vi "Generate Rectangle Seq Img Core.vi"(6 "TDMS file path & name":path=path "C:/Users/Theo/Desktop/Datasets/140401_17_44_08-rig 3 debugging/Functional imaging TDMS data files/001.tdms", 7 "Channel to process":enum16{"Red", "Green"}(ring), 8 "error in (no error)":errorcluster, 9 "<Vol images/video folder>":path, 10 "All header parameters":T1={"LOGIN"={"User"="Olympus  20X", "Profile"="", "Software Version"="", "Experiment Date Time"=timestamp(0 s since 1904-01-01)}, "GLOBAL PARAMETERS"={"MicroscopeID"="", "Microscope Type"="", "Objective"="", "Field of View (um)"=0.0, "Fill time (us)"=0.0, "Experiment Type"=enum."In vivo", "Stimuli Trigger"=FALSE, "Speed Logging"=FALSE}, "IMAGING MODES"={"Time Series"=FALSE, "Motor Zstack"=FALSE, "AOL Zstack"=FALSE, "Functional Imaging"=FALSE, "Volume Imaging"=FALSE}, "TIME SERIES"={"Basic Image meta data"={"Wavelength (nm)"=0.0, "# averaged frames"=0.0, "laser power (%)"=0.0, "Pockels"=0.0, "pixel dwell time (us)"=0.0, "pmt 1"=0.0, "pmt 2"=0.0, "back apperture"=0.0, "zoom"=0.0, "field of view"=0.0, "Frame Size"=0, "AOL x centre"=200.0, "AOL y centre"=0.0, "Stage x position"=0.0, "Stage y position"=0.0, "Stage z position"=0.0}, "AOL z"=0.0}, "MOTOR Z-STACK "={"Hdr Basic Image meta data"={"Wavelength (nm)"=0.0, "# averaged frames"=0.0, "laser power (%)"=0.0, "Pockels"=0.0, "pixel dwell time (us)"=0.0, "pmt 1"=0.0, "pmt 2"=0.0, "back apperture"=0.0, "zoom"=0.0, "field of view"=0.0, "Frame Size"=0, "AOL x centre"=0.0, "AOL y centre"=0.0, "Stage x position"=0.0, "Stage y position"=0.0, "Stage z position"=0.0}, "Z Start"=0.0, "Z Stop"=0.0, "No of Planes"=0}, "AOL Z-STACK"={"Hdr Basic Image meta data"={"Wavelength (nm)"=0.0, "# averaged frames"=0.0, "laser power (%)"=0.0, "Pockels"=0.0, "pixel dwell time (us)"=0.0, "pmt 1"=0.0, "pmt 2"=0.0, "back apperture"=0.0, "zoom"=0.0, "field of view"=0.0, "Frame Size"=0, "AOL x centre"=0.0, "AOL y centre"=0.0, "Stage x position"=0.0, "Stage y position"=0.0, "Stage z position"=0.0}, "Z Start"=0.0, "Z Stop"=0.0, "No of Planes"=0}, "FUNCTIONAL IMAGING"={"Functional Mode"=enum."Point", "Pockels Modulation"=FALSE, "Number of pois"=0.0, "Number of miniscans"=0.0, "Number of cycles"=0.0, "Number of trials"=0.0, "Miniscan dwell time per pixel (us)"=0.0, "Number of pixels in miniscan"=0.0, "poi dwell time"=0.0, "Rectangle ROI length"=0.0, "Rectangle ROI height"=0.0, "AOL Mode"=enum."Raster", "Plane Mode"=0, "video length (sec)"=0.0, "Frame rate (fps)"=0.0, "Stimuli Timing (usec)"=0.0, "Acquisition Length"=0.0, "Basic Image meta data"={"Wavelength (nm)"=0.0, "# averaged frames"=0.0, "laser power (%)"=0.0, "Pockels"=0.0, "pixel dwell time (us)"=0.0, "pmt 1"=0.0, "pmt 2"=0.0, "back apperture"=0.0, "zoom"=0.0, "field of view"=0.0, "Frame Size"=0, "AOL x centre"=0.0, "AOL y centre"=0.0, "Stage x position"=0.0, "Stage y position"=0.0, "Stage z position"=0.0}, "Z Start (um)"=0.0, "Z Stop (um)"=0.0}, "VOLUME IMAGING"={"Functional Mode"=enum."Point", "Pockels Modulation"=FALSE, "Number of pois"=0.0, "Number of miniscans"=0.0, "Number of cycles"=0.0, "Number of trials"=0.0, "Miniscan dwell time per pixel (us)"=0.0, "Number of pixels in miniscan"=0.0, "poi dwell time"=0.0, "Rectangle ROI length"=0.0, "Rectangle ROI height"=0.0, "AOL Mode"=enum."Raster", "Plane Mode"=0, "video length (sec)"=0.0, "Frame rate (fps)"=0.0, "Stimuli Timing (usec)"=0.0, "Acquisition Length"=0.0, "Basic Image meta data"={"Wavelength (nm)"=0.0, "# averaged frames"=0.0, "laser power (%)"=0.0, "Pockels"=0.0, "pixel dwell time (us)"=0.0, "pmt 1"=0.0, "pmt 2"=0.0, "back apperture"=0.0, "zoom"=0.0, "field of view"=0.0, "Frame Size"=0, "AOL x centre"=0.0, "AOL y centre"=0.0, "Stage x position"=0.0, "Stage y position"=0.0, "Stage z position"=0.0}, "Z Start (um)"=0.0, "Z Stop (um)"=0.0}, "CALIBRATION"={"Pockels Calibration File"=path "", "Calibration_ini file"=path "", "Setup_ini file"=path ""}, "STATISTICS"={"Z-stack duration (sec)"=0.0, "Number of acquired data-points"=0.0, "Acquisition time (ms)"=0.0, "Number of acquired frames"=0.0, "Intertrial times"=[]}, "BIOLOGY INFORMATION"={"Animal Code or Name"="", "Animal DoB"="", "Animal Age"="", "Animal Sex"="", "Animal Weight"="", "Date of Injection"="", "Date of Implant"="", "Site of Injection"="", "Animal Ear Notch"="", "AAV constructs"="", "Genetic background"="", "Optical reporter"="", "Region of brain imaged"="", "Other \ncomments"=""}} {"VOLUME IMAGING"."Plane Mode" items=["XY Plane", "XZ Plane", "YZ Plane", "arbitraryplane"]; "VOLUME IMAGING"."Basic Image meta data"."Frame Size" items=["100X100"=100, "128X128"=128, "200X200"=200, "256X256"=256, "512X512"=512, "1024x1024"=1024, "2048x2048"=2048]; "AOL Z-STACK"."Hdr Basic Image meta data"."Frame Size" items=["100X100"=100, "128X128"=128, "200X200"=200, "256X256"=256, "512X512"=512, "1024x1024"=1024, "2048x2048"=2048]; "MOTOR Z-STACK"."Hdr Basic Image meta data"."Frame Size" items=["100X100"=100, "128X128"=128, "200X200"=200, "256X256"=256, "512X512"=512, "1024x1024"=1024, "2048x2048"=2048]; "FUNCTIONAL IMAGING"."Plane Mode" items=["XY Plane", "XZ Plane", "YZ Plane", "arbitraryplane"]; "FUNCTIONAL IMAGING"."Basic Image meta data"."Frame Size" items=["100X100"=100, "128X128"=128, "200X200"=200, "256X256"=256, "512X512"=512, "1024x1024"=1024, "2048x2048"=2048]; "TIME SERIES"."Basic Image meta data"."Frame Size" items=["100X100"=100, "128X128"=128, "200X200"=200, "256X256"=256, "512X512"=512, "1024x1024"=1024, "2048x2048"=2048]}, 11 "tdms file ref":refnum<k34>) -> (0 "error out":errorcluster, 3 "tdms file out":refnum<k34>)   [LabVIEW 2017]
uses:
  User Interface/Visualisation/Functional Imaging Viewer/SubVIs/Experiment header interface/Typedefs/Header parameters cluster-ALL.ctl
  User Interface/Visualisation/Functional Imaging Viewer/SubVIs/Experiment header interface/Typedefs/Header subclusters/Header params -Login.ctl
  User Interface/Visualisation/Functional Imaging Viewer/SubVIs/Experiment header interface/Typedefs/Header subclusters/Header params-Global Parameters.ctl
  User Interface/Misc/Experiment Type.ctl
  User Interface/Visualisation/Functional Imaging Viewer/SubVIs/Experiment header interface/Typedefs/Header subclusters/Header params-Imaging Modes.ctl
  User Interface/Visualisation/Functional Imaging Viewer/SubVIs/Experiment header interface/Typedefs/Header subclusters/Header params-Time Series.ctl
  User Interface/Visualisation/Functional Imaging Viewer/SubVIs/Experiment header interface/Typedefs/Header subclusters/Header params-Basic image meta data.ctl
  Typedefs/Frame Size.ctl
  User Interface/Visualisation/Functional Imaging Viewer/SubVIs/Experiment header interface/Typedefs/Header subclusters/Header params-Motor Z-stack.ctl
  User Interface/Visualisation/Functional Imaging Viewer/SubVIs/Experiment header interface/Typedefs/Header subclusters/Header params-AOL Z-stack.ctl
  User Interface/Visualisation/Functional Imaging Viewer/SubVIs/Experiment header interface/Typedefs/Header subclusters/Header params-Functional Imaging.ctl
  Typedefs/Functional Mode.ctl
  Typedefs/AOL modes.ctl
  Typedefs/Plane Mode.ctl
  User Interface/Visualisation/Functional Imaging Viewer/SubVIs/Experiment header interface/Typedefs/Header subclusters/Header params-Calibration Setup.ctl
  User Interface/Visualisation/Functional Imaging Viewer/SubVIs/Experiment header interface/Typedefs/Header subclusters/Header params-statistics.ctl
  User Interface/Misc/Biology Information.ctl
  Typedefs/Channel Selector.ctl
  <vilib>/vision/NI_Vision_Development_Module.lvlib
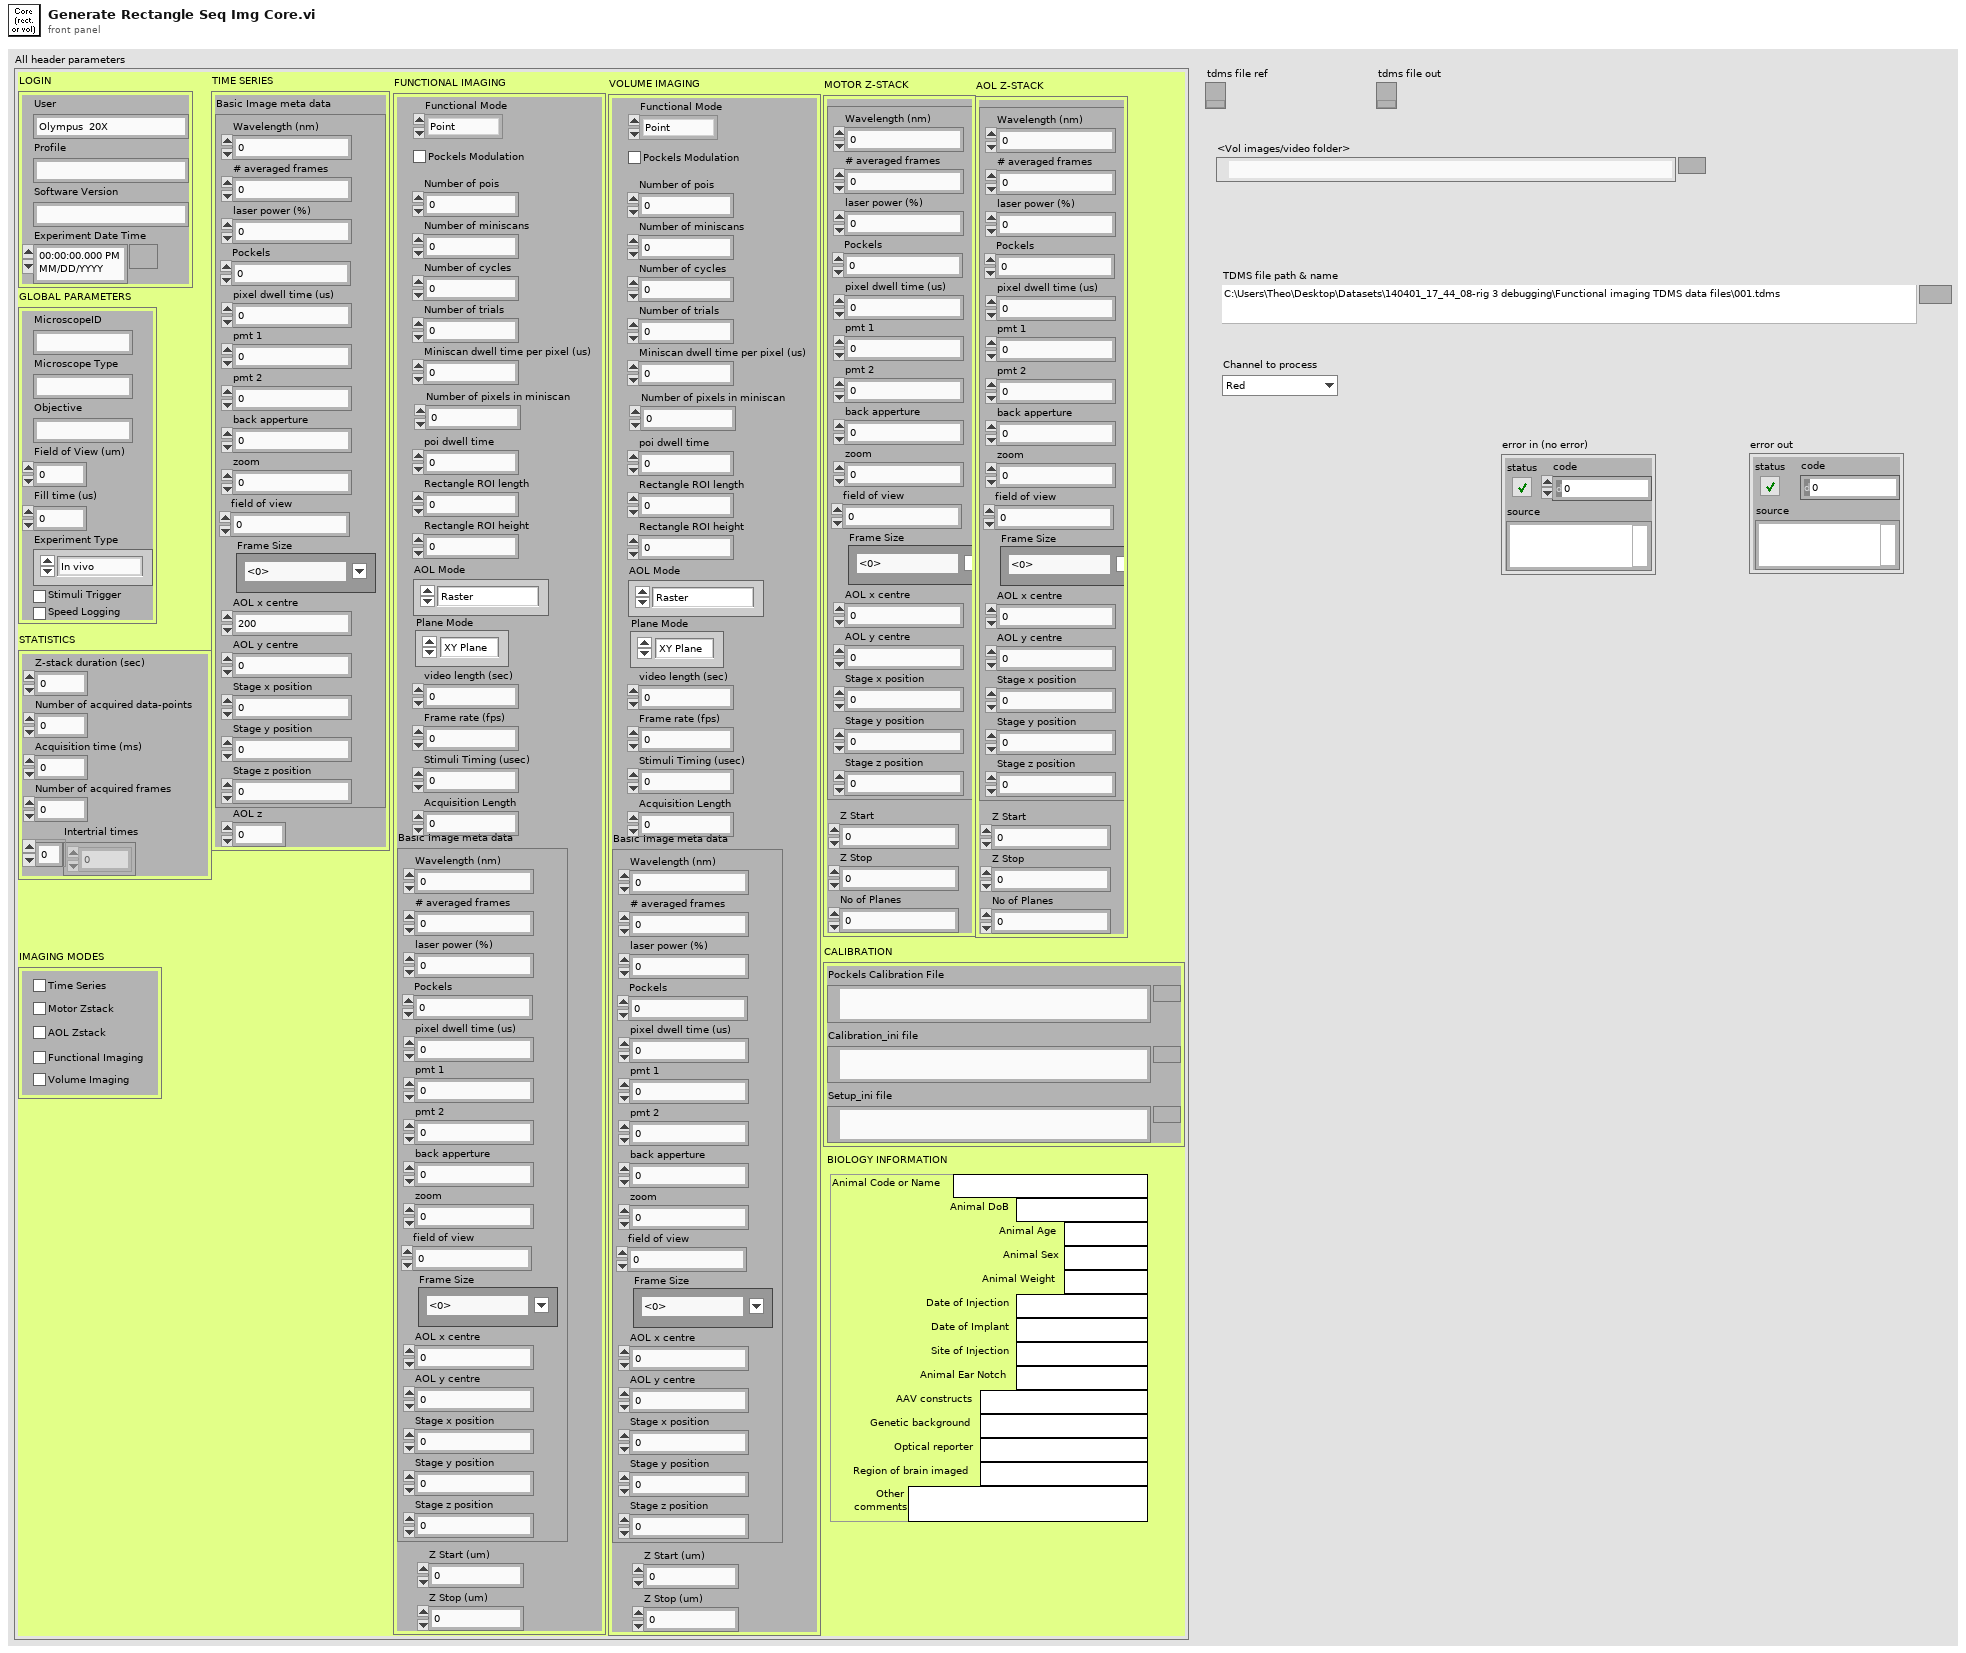
[diagram p1: front panel]
types:
  T1 = typedef "Header parameters cluster-ALL.ctl" = cluster{"LOGIN":T2, "GLOBAL PARAMETERS":T3, "IMAGING MODES":T5, "TIME SERIES":T6, "MOTOR Z-STACK ":T9, "AOL Z-STACK":T10, "FUNCTIONAL IMAGING":T11, "VOLUME IMAGING":T11, "CALIBRATION":T15, "STATISTICS":T16, "BIOLOGY INFORMATION":T17}
  T2 = typedef "Header params -Login.ctl" = cluster{"User":string, "Profile":string, "Software Version":string, "Experiment Date Time":timestamp}
  T3 = typedef "Header params-Global Parameters.ctl" = cluster{"MicroscopeID":string, "Microscope Type":string, "Objective":string, "Field of View (um)":dbl, "Fill time (us)":dbl, "Experiment Type":T4, "Stimuli Trigger":bool, "Speed Logging":bool}
  T4 = typedef "Experiment Type.ctl" = enum16{"In vivo", "In vitro", "Testing", "Calibration", "Other"}
  T5 = typedef "Header params-Imaging Modes.ctl" = cluster{"Time Series":bool, "Motor Zstack":bool, "AOL Zstack":bool, "Functional Imaging":bool, "Volume Imaging":bool}
  T6 = typedef "Header params-Time Series.ctl" = cluster{"Basic Image meta data":T7, "AOL z":dbl}
  T7 = typedef "Header params-Basic image meta data.ctl" = cluster{"Wavelength (nm)":dbl, "# averaged frames":dbl, "laser power (%)":dbl, "Pockels":dbl, "pixel dwell time (us)":dbl, "pmt 1":dbl, "pmt 2":dbl, "back apperture":dbl, "zoom":dbl, "field of view":dbl, "Frame Size":T8, "AOL x centre":dbl, "AOL y centre":dbl, "Stage x position":dbl, "Stage y position":dbl, "Stage z position":dbl}
  T8 = typedef "Frame Size.ctl" = u16
  T9 = typedef "Header params-Motor Z-stack.ctl" = cluster{"Hdr Basic Image meta data":T7, "Z Start":dbl, "Z Stop":dbl, "No of Planes":i32}
  T10 = typedef "Header params-AOL Z-stack.ctl" = cluster{"Hdr Basic Image meta data":T7, "Z Start":dbl, "Z Stop":dbl, "No of Planes":i32}
  T11 = typedef "Header params-Functional Imaging.ctl" = cluster{"Functional Mode":T12, "Pockels Modulation":bool, "Number of pois":dbl, "Number of miniscans":dbl, "Number of cycles":dbl, "Number of trials":dbl, "Miniscan dwell time per pixel (us)":dbl, "Number of pixels in miniscan":dbl, "poi dwell time":dbl, "Rectangle ROI length":dbl, "Rectangle ROI height":dbl, "AOL Mode":T13, "Plane Mode":T14, "video length (sec)":dbl, "Frame rate (fps)":dbl, "Stimuli Timing (usec)":dbl, "Acquisition Length":dbl, "Basic Image meta data":T7, "Z Start (um)":dbl, "Z Stop (um)":dbl}
  T12 = typedef "Functional Mode.ctl" = enum16{"Point", "Line", "Patch", "Plane", "Volume"}
  T13 = typedef "AOL modes.ctl" = enum16{"Raster", "Structural", "Pointing", "Mini Scan", "Alignment"}
  T14 = typedef "Plane Mode.ctl" = u16
  T15 = typedef "Header params-Calibration Setup.ctl" = cluster{"Pockels Calibration File":path, "Calibration_ini file":path, "Setup_ini file":path}
  T16 = typedef "Header params-statistics.ctl" = cluster{"Z-stack duration (sec)":dbl, "Number of acquired data-points":dbl, "Acquisition time (ms)":dbl, "Number of acquired frames":dbl, "Intertrial times":dbl[]}
  T17 = typedef "Biology Information.ctl" = cluster{"Animal Code or Name":string, "Animal DoB":string, "Animal Age":string, "Animal Sex":string, "Animal Weight":string, "Date of Injection":string, "Date of Implant":string, "Site of Injection":string, "Animal Ear Notch":string, "AAV constructs":string, "Genetic background":string, "Optical reporter":string, "Region of brain imaged":string, "Other \ncomments":string}
  T18 = typedef "Channel Selector.ctl" = enum16{"Red Channel", "Green Channel", "Blended"}
  T19 = cluster{"Number of cycles":i32, "number of planes":i32, "number of miniscans in a Plane":i32, "number of pixels in a miniscan":i32}
  T20 = typedef "Image Type" = u32
  T21 = typedef "IMAQ Image.ctl" = refnum<image>
  T22 = typedef "IMAQ AVI2 Refnum.ctl" = refnum<k20>
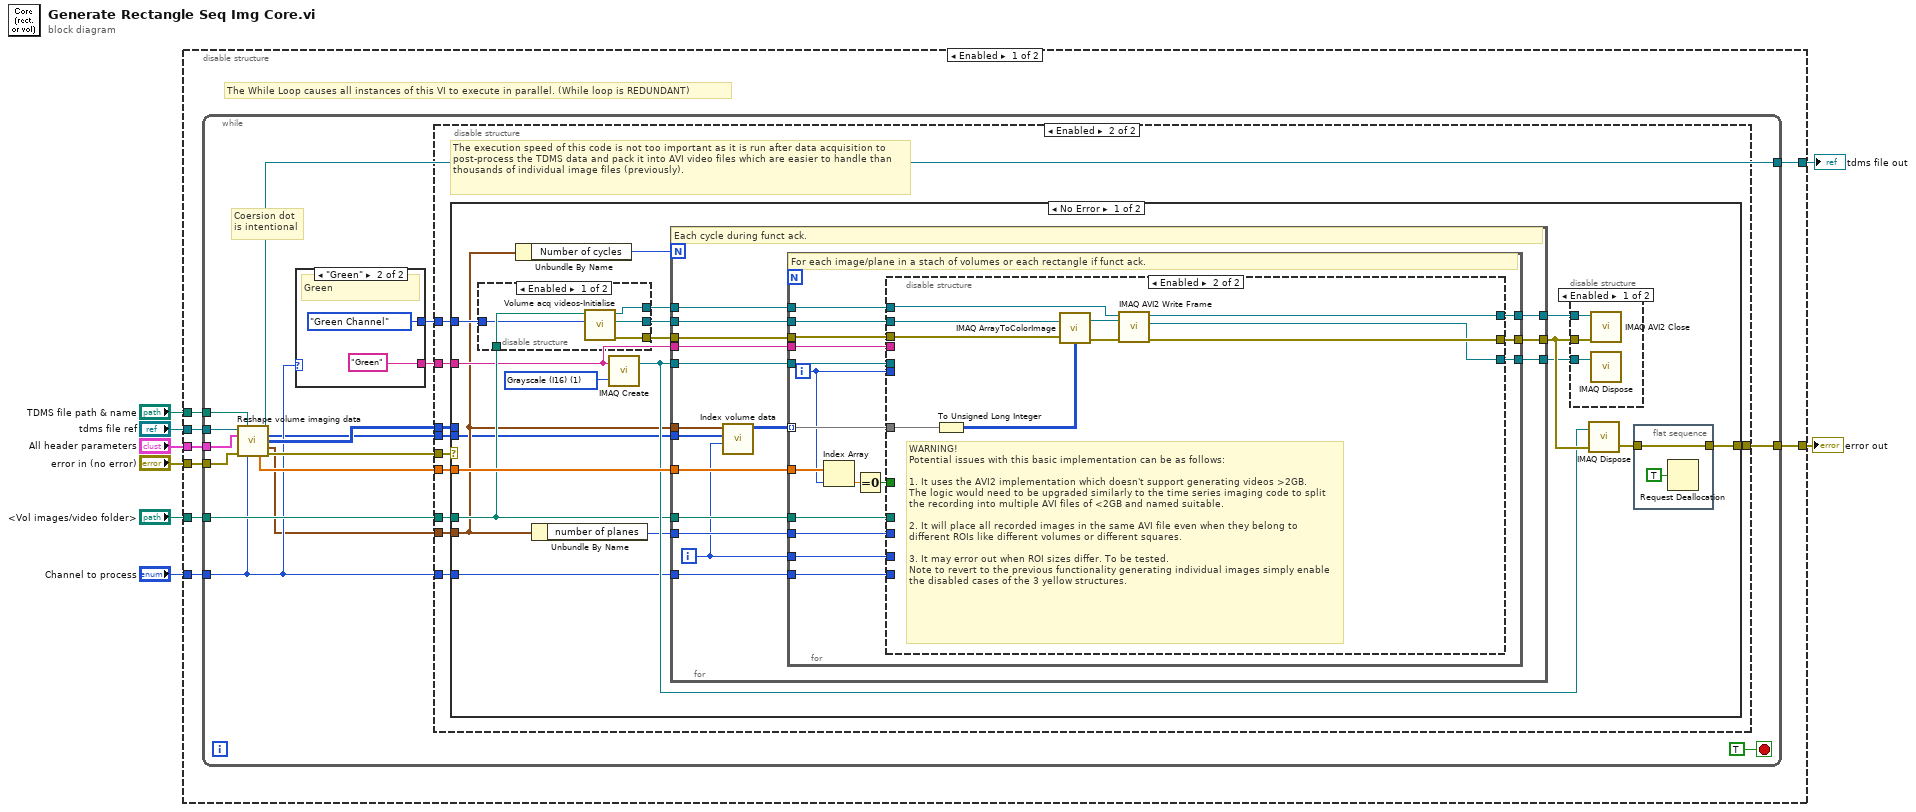
[diagram p0: block diagram]
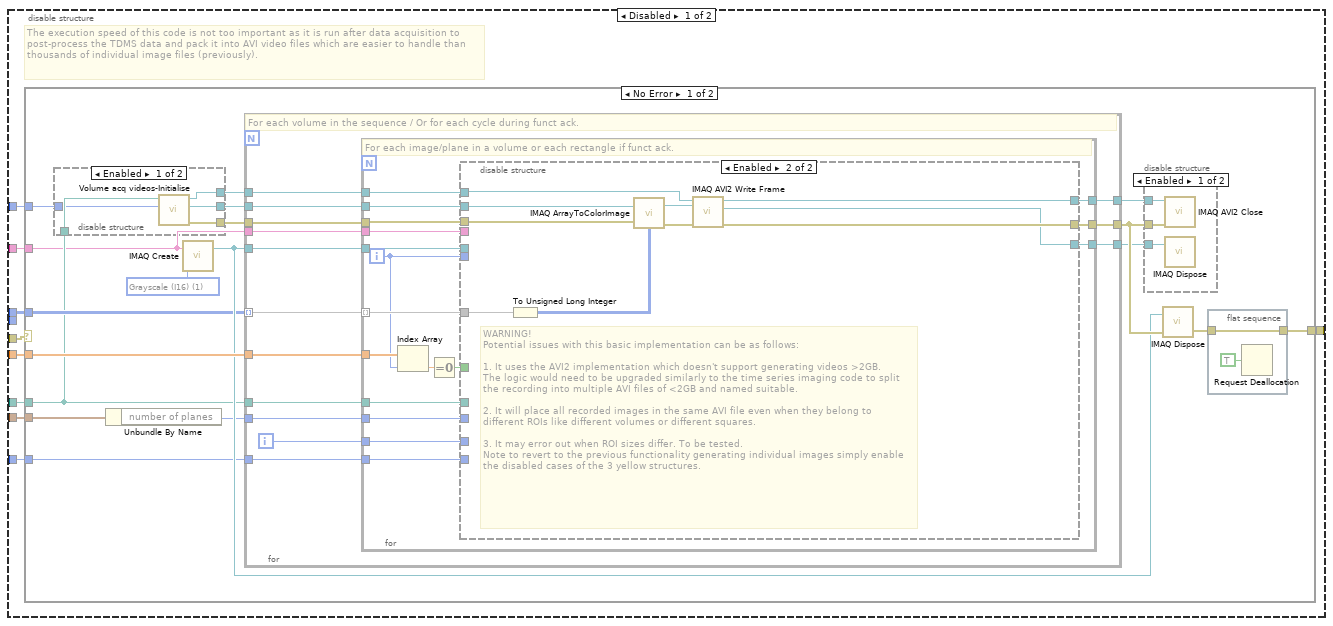
[diagram p2: hidden frame]
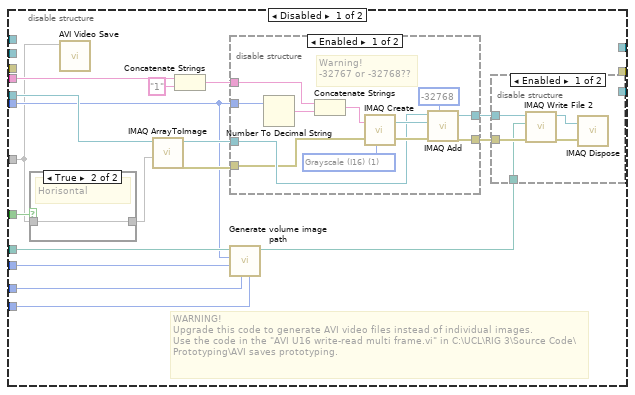
[diagram p5: hidden frame]
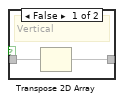
[diagram p6: hidden frame]
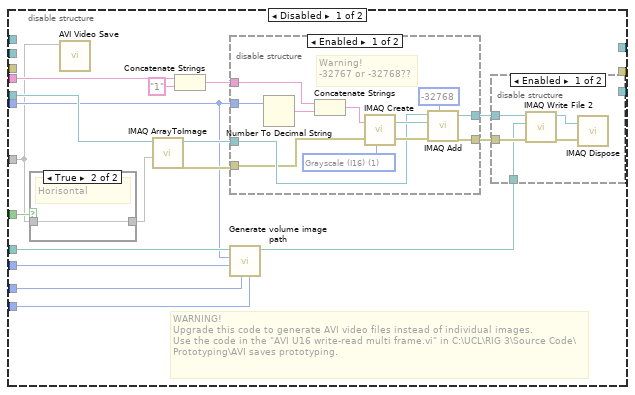
[diagram p12: hidden frame]
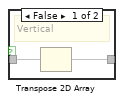
[diagram p13: hidden frame]
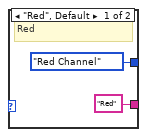
[diagram p17: hidden frame]
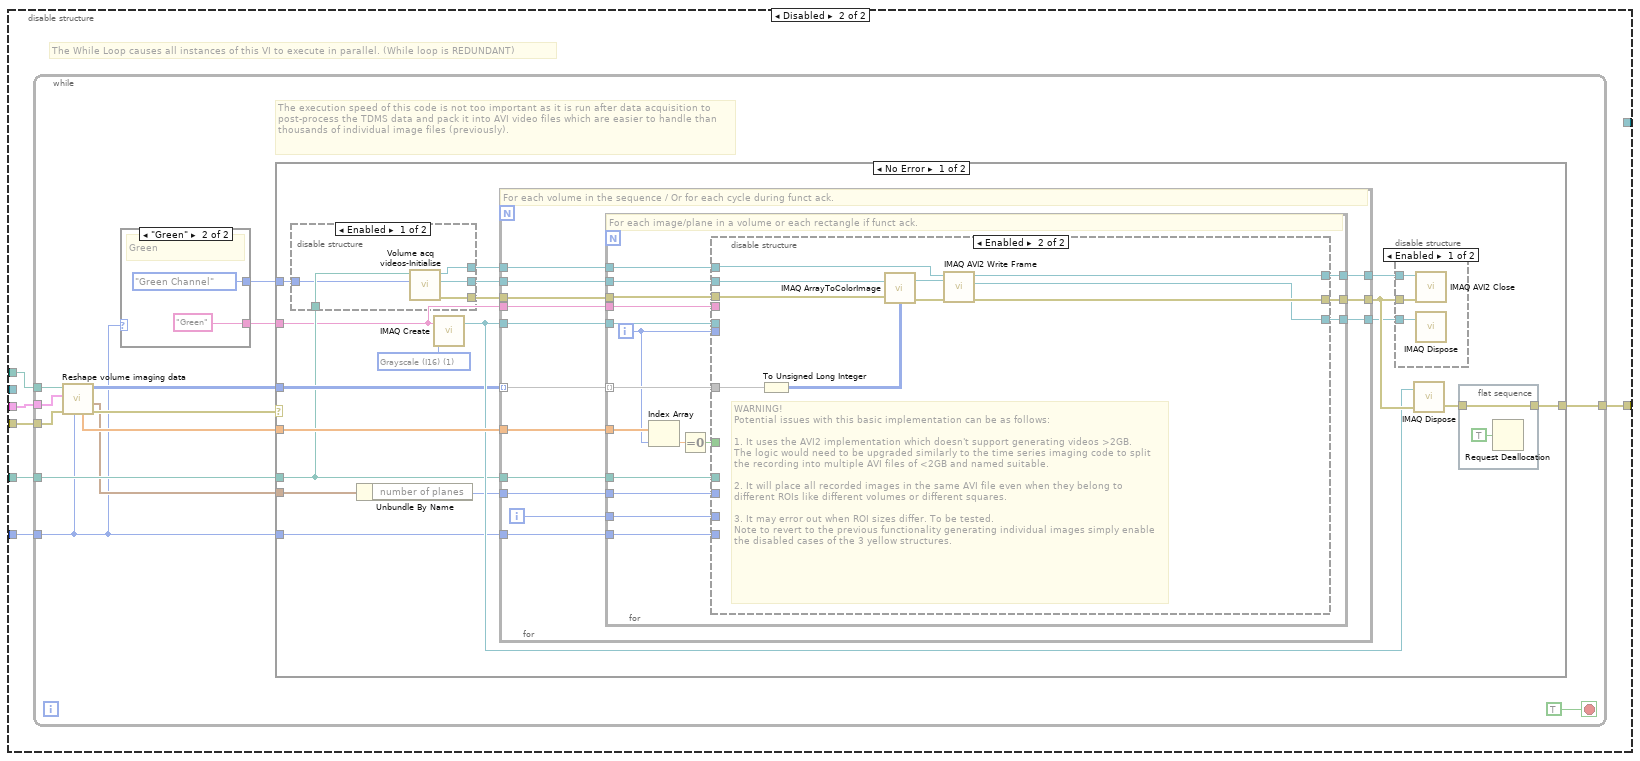
[diagram p18: hidden frame]
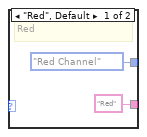
[diagram p19: hidden frame]
diagram:
  n1 = disable-structure shown="Enabled" {
    disable-tunnel: [w16 w282] -> w8
    disable-tunnel: "<Vol images/video folder>" -> [w15 w281]
    disable-tunnel: "TDMS file path & name" -> [w14 w280]
    disable-tunnel: "error in (no error)" -> [w13 w279]
    disable-tunnel: "All header parameters" -> [w12 w278]
    disable-tunnel: "Channel to process" -> [w11 w277]
    disable-tunnel: "tdms file ref" -> [w10 _]
    disable-tunnel: [w9 _] -> w1
    frame Enabled {
      # "The While Loop causes all instances of this VI to execute in parallel. (While loop is REDUNDANT)"
      n2 = while {
        tunnel: [w32] -> w16
        tunnel: w15 -> [w31]
        tunnel: w14 -> [w30]
        tunnel: w11 -> [w21]
        tunnel: w13 -> [w26]
        tunnel: w12 -> [w23]
        tunnel: w10 -> [w18]
        tunnel: [w17] -> w9
        stop <- TRUE stop-if-true
        # "Coersion dot\nis intentional"
        n3 = call "Reshape volume imaging data.vi"("tdms file ref"=w18, "TDMS file path & name"=w30, "All header parameters"=w23, "error in (no error)"=w26, "Channel to process"=w21) -> ("tdms file out"=w17:refnum<k34>, "Single channel data"=w19:u16[], "Channel 4D data"=w28:u16[][][][], "Volumetric parameters"=w20:T19, "Angles (deg)"=w22:dbl[], "error out"=w27:errorcluster)  [unwired: 5 in]
        n4 = case shown="\"Green\"" w21 {
          tunnel: ["Red" ("Image Name") "Green" ("Image Name")] -> w29
          tunnel: [Channel_Selector."Red Channel" ("Channel") Channel_Selector."Green Channel" ("Channel")] -> w25
          frame "Red", Default {
            # "Red"
          }
          frame "Green" {
            # "Green"
          }
        }
        n5 = disable-structure shown="Enabled" {
          disable-tunnel: [w41 w160] -> w32
          disable-tunnel: w31 -> [w40 w159]
          disable-tunnel: w29 -> [w39 w158]
          disable-tunnel: w28 -> [w38 w157]
          disable-tunnel: w27 -> [w37 w156]
          disable-tunnel: w25 -> [w36 w155]
          disable-tunnel: w22 -> [w35 w154]
          disable-tunnel: w21 -> [w34 w153]
          disable-tunnel: w20 -> [w33 w152]
          disable-tunnel: w19 -> [_ w151]
          frame Disabled {
            # "The execution speed of this code is not too important as it is run after data acquisition to post-process the TDMS data and pack it into AVI video files which are easier to handle than thousands of individual image files (previously)."
            n6 = case shown="No Error" w37 {
              selector: w37 -> [_ w150]
              tunnel: [w45 w150] -> w41
              tunnel: w35 -> [w59 _]
              tunnel: w38 -> [w51 _]
              tunnel: w33 -> [w42 _]
              tunnel: w40 -> [w48 _]
              tunnel: w39 -> [w47 _]
              tunnel: w34 -> [w44 _]
              tunnel: w36 -> [w43 _]
              frame No Error {
                w50 = T20 1 items=["Grayscale (U8)", "Grayscale (I16)", "Grayscale (SGL)", "Complex (CSG)", "RGB (U32)", "HSL (U32)", "RGB (U64)", "Grayscale (U16)"] ("Image Type")
                n7 = disable-structure "Diagram Disable Structure" shown="Enabled" {
                  disable-tunnel: [w66 _] -> w52
                  disable-tunnel: [w65 _] -> w53
                  disable-tunnel: [w64 _] -> w54
                  disable-tunnel: w48 -> [w63 _]
                  disable-tunnel: w43 -> [w62 _]
                  frame Enabled {
                    n8 = call "Volume acq videos-Initialise.vi"("Channel"=w62, "created path"=w63) -> ("error out"=w66:errorcluster, "Temp Image"=w65:T21, "Refnum out"=w64:T22)  [unwired: 7 in]
                  }
                  frame Disabled {
                  }
                }
                n9 = Unbundle By Name(w42) -> ("number of planes"=w49:i32)
                n10 = call "IMAQ Create"("Image Name"=w47, "Image Type"=w50) -> ("New Image"=w57:T21)  [unwired: 3 in, 1 out]
                n11 = for {
                  tunnel: w51 -> [w83] mode=indexing
                  tunnel: w57 -> [w82]
                  tunnel: w48 -> [w81]
                  tunnel: w49 -> [w79]
                  tunnel: w53 -> [w78]
                  tunnel: w54 -> [w77]
                  tunnel: w52 -> [w76]
                  tunnel: [w75] -> w58
                  tunnel: [w74] -> w55
                  tunnel: [w73] -> w56
                  tunnel: w59 -> [w72]
                  tunnel: w47 -> [w71]
                  tunnel: w44 -> [w70]
                  i -> [w80]
                  # "For each volume in the sequence / Or for each cycle during funct ack."
                  n12 = for {
                    tunnel: w83 -> [w87] mode=indexing
                    tunnel: w82 -> [w100]
                    tunnel: w81 -> [w99]
                    tunnel: w80 -> [w98]
                    tunnel: w79 -> [w97]
                    tunnel: w78 -> [w95]
                    tunnel: w77 -> [w96]
                    tunnel: w76 -> [w94]
                    tunnel: [w93] -> w75
                    tunnel: [w92] -> w74
                    tunnel: [w91] -> w73
                    tunnel: w72 -> [w86]
                    tunnel: w71 -> [w89]
                    tunnel: w70 -> [w88]
                    i -> [w85]
                    # "For each image/plane in a volume or each rectangle if funct ack."
                    n13 = Index Array(array=w86, index=w85) -> (element=w84:dbl)
                    n14 = Equal To 0?(x=w84) -> (x = 0?=w90:bool)
                    n15 = disable-structure shown="Enabled" {
                      disable-tunnel: w100 -> [w117 _]
                      disable-tunnel: w99 -> [w112 _]
                      disable-tunnel: w98 -> [w110 _]
                      disable-tunnel: w97 -> [w109 _]
                      disable-tunnel: w85 -> [w108 _]
                      disable-tunnel: w96 -> [_ w146]
                      disable-tunnel: w95 -> [_ w145]
                      disable-tunnel: w94 -> [_ w144]
                      disable-tunnel: [_ w143] -> w93
                      disable-tunnel: [_ w142] -> w92
                      disable-tunnel: [_ w141] -> w91
                      disable-tunnel: w90 -> [w107 _]
                      disable-tunnel: w87 -> [w102 w140]
                      disable-tunnel: w89 -> [w105 _]
                      disable-tunnel: w88 -> [w101 _]
                      frame Disabled {
                        # "WARNING!\nUpgrade this code to generate AVI video files instead of individual images.\nUse the code in the \"AVI U16 write-read multi frame.vi\" in C:\\UCL\\RIG 3\\Source Code\\Prototyping\\AVI saves prototyping."
                        n16 = case shown="True" w107 {
                          tunnel: w102 -> [w119 w120]
                          tunnel: [w118 w120] -> w106
                          frame False {
                            # "Vertical"
                            n17 = Transpose 2D Array(2D array=w119) -> (transposed array=w118:u16[][])
                          }
                          frame True {
                            # "Horisontal"
                          }
                        }
                        n18 = call "AVI Video Save.vi"("Image Pixels"=w102) -> ()  [unwired: 9 in, 2 out]
                        n19 = call "IMAQ ArrayToImage"("Image Pixels (I16)"=w106, "Image"=w117) -> ("error out"=w113:errorcluster, "Image Out"=w116:T21)  [unwired: 8 in]
                        n20 = Concatenate Strings(w105, "1" ("string")) -> (w103:string)
                        n21 = call "Generate volume image path.vi"("Channel to process"=w101, "Volume index"=w110, "Number of planes"=w109, "Plane index (within its volume)"=w108, "Folder path"=w112) -> ("File path"=w111:path)  [unwired: 5 in, 1 out]
                        n22 = disable-structure shown="Enabled" {
                          disable-tunnel: w108 -> [w131 _]
                          disable-tunnel: w116 -> [w130 w139]
                          disable-tunnel: [w129 w139] -> w115
                          disable-tunnel: [w127 w138] -> w114
                          disable-tunnel: w113 -> [w128 w138]
                          disable-tunnel: w103 -> [w126 _]
                          frame Enabled {
                            w133 = T20 1 items=["Grayscale (U8)", "Grayscale (I16)", "Grayscale (SGL)", "Complex (CSG)", "RGB (U32)", "HSL (U32)", "RGB (U64)"] ("Image Type")
                            # "Warning!\n-32767 or -32768??"
                            n23 = Number To Decimal String(number=w131) -> (decimal integer string=w134:string)  [unwired: 1 in]
                            n24 = Concatenate Strings(w126, w134) -> (w135:string)
                            n25 = call "IMAQ Create"("Image Name"=w135, "Image Type"=w133, "error in (no error)"=w128) -> ("New Image"=w136:T21, "error out"=w137:errorcluster)  [unwired: 2 in]
                            n26 = call "IMAQ Add"("Image Src A"=w130, "Constant"=i16 -32768, "Image Dst"=w136, "error in (no error)"=w137) -> ("Image Dst Out"=w129:T21, "error out"=w127:errorcluster)  [unwired: 3 in]
                          }
                          frame Disabled {
                          }
                        }
                        n27 = disable-structure shown="Enabled" {
                          disable-tunnel: w115 -> [w123 _]
                          disable-tunnel: w114 -> [w122 _]
                          disable-tunnel: w111 -> [w121 _]
                          frame Enabled {
                            n28 = call-poly "IMAQ Write File 2"("error in (no error)"=w122, "File Path"=w121, "Image"=w123) -> ("error out"=w125:errorcluster, "Image Out (duplicate)"=w124:T21)  [unwired: 7 in]
                            n29 = call "IMAQ Dispose"("Image"=w124, "error in (no error)"=w125) -> ()  [unwired: 4 in, 1 out]
                          }
                          frame Disabled {
                          }
                        }
                      }
                      frame Enabled {
                        # "WARNING!\nPotential issues with this basic implementation can be as follows:\n\n1. It uses the AVI2 implementation which doesn't support generating videos >2GB. \nThe logic would need to be upgraded similarly to the time series imaging code to split the recording into multiple AVI files of <2GB and named suitable.\n\n2. It will place all recorded images in the same AVI file even when they belong to different ROIs like different volumes or different squares.\n\n3. It may error out when ROI sizes differ. To be tested.\nNote to revert to the previous functionality generating individual images simply enable the disabled cases of the 3 yellow structures."
                        n30 = To Unsigned Long Integer(number=w140) -> (unsigned 32bit integer=w148:u32[][])
                        n31 = call "IMAQ ArrayToColorImage"("Image Pixels (U32)"=w148, "Image"=w145, "error in (no error)"=w144) -> ("Image Out"=w149:T21, "error out"=w147:errorcluster)  [unwired: 1 in, 1 out]
                        n32 = call "IMAQ AVI2 Write Frame"("error in (no error)"=w147, "Image"=w149, "AVI Refnum"=w146) -> ("error out"=w143:errorcluster, "Image Out (duplicate)"=w141:T21, "AVI Refnum (duplicate)"=w142:T22)  [unwired: 6 in]
                      }
                    }
                  }
                }
                n33 = disable-structure "Diagram Disable Structure" shown="Enabled" {
                  disable-tunnel: w55 -> [w69 _]
                  disable-tunnel: w58 -> [w68 _]
                  disable-tunnel: w56 -> [w67 _]
                  frame Enabled {
                    n34 = call "IMAQ AVI2 Close"("error in (no error)"=w68, "AVI Refnum"=w69) -> ()  [unwired: 9 in, 1 out]
                    n35 = call "IMAQ Dispose"("Image"=w67) -> ()  [unwired: 5 in, 1 out]
                  }
                  frame Disabled {
                  }
                }
                n36 = call "IMAQ Dispose"("Image"=w57, "error in (no error)"=w58) -> ("error out"=w46:errorcluster)  [unwired: 4 in]
                n37 = flat-sequence {
                  tunnel: w46 -> [w60]
                  tunnel: [w60] -> w45
                  frame #0 {
                    n38 = Request Deallocation(TRUE ("flag")) -> ()
                  }
                }
              }
              frame Error {
              }
            }
          }
          frame Enabled {
            # "The execution speed of this code is not too important as it is run after data acquisition to post-process the TDMS data and pack it into AVI video files which are easier to handle than thousands of individual image files (previously)."
            n39 = case shown="No Error" w156 {
              selector: w156 -> [_ w272]
              tunnel: [w166 w272] -> w160
              tunnel: w154 -> [w179 _]
              tunnel: w157 -> [_ _]
              tunnel: w152 -> [w162 _]
              tunnel: w159 -> [w169 _]
              tunnel: w158 -> [w168 _]
              tunnel: w153 -> [w165 _]
              tunnel: w155 -> [w164 _]
              tunnel: w151 -> [w161 _]
              frame No Error {
                w171 = T20 1 items=["Grayscale (U8)", "Grayscale (I16)", "Grayscale (SGL)", "Complex (CSG)", "RGB (U32)", "HSL (U32)", "RGB (U64)", "Grayscale (U16)"] ("Image Type")
                n40 = disable-structure "Diagram Disable Structure" shown="Enabled" {
                  disable-tunnel: [w186 _] -> w172
                  disable-tunnel: [w185 _] -> w173
                  disable-tunnel: [w184 _] -> w174
                  disable-tunnel: w169 -> [w183 _]
                  disable-tunnel: w164 -> [w182 _]
                  frame Enabled {
                    n41 = call "Volume acq videos-Initialise.vi"("Channel"=w182, "created path"=w183) -> ("error out"=w186:errorcluster, "Temp Image"=w185:T21, "Refnum out"=w184:T22)  [unwired: 7 in]
                  }
                  frame Disabled {
                  }
                }
                n42 = Unbundle By Name(w162) -> ("Number of cycles"=w163:i32)
                n43 = Unbundle By Name(w162) -> ("number of planes"=w170:i32)
                n44 = call "IMAQ Create"("Image Name"=w168, "Image Type"=w171) -> ("New Image"=w177:T21)  [unwired: 3 in, 1 out]
                n45 = for {
                  N: w163 -> [_]
                  tunnel: w177 -> [w205]
                  tunnel: w169 -> [w204]
                  tunnel: w170 -> [w203]
                  tunnel: w173 -> [w202]
                  tunnel: w174 -> [w201]
                  tunnel: w172 -> [w200]
                  tunnel: [w199] -> w178
                  tunnel: [w198] -> w175
                  tunnel: [w197] -> w176
                  tunnel: w179 -> [w196]
                  tunnel: w168 -> [w195]
                  tunnel: w165 -> [w194]
                  tunnel: w162 -> [w192]
                  tunnel: w161 -> [w191]
                  i -> [w190]
                  # "Each cycle during funct ack."
                  n46 = call "Index volume data.vi"("Cycle index"=w190, "Single trial data (single channel)"=w191, "Parameters Cluster"=w192) -> ("3D"=w193:u16[][][])  [unwired: 5 in, 3 out]
                  n47 = for {
                    tunnel: w193 -> [w209] mode=indexing
                    tunnel: w205 -> [w222]
                    tunnel: w204 -> [w221]
                    tunnel: w190 -> [w220]
                    tunnel: w203 -> [w219]
                    tunnel: w202 -> [w217]
                    tunnel: w201 -> [w218]
                    tunnel: w200 -> [w216]
                    tunnel: [w215] -> w199
                    tunnel: [w214] -> w198
                    tunnel: [w213] -> w197
                    tunnel: w196 -> [w208]
                    tunnel: w195 -> [w211]
                    tunnel: w194 -> [w210]
                    i -> [w207]
                    # "For each image/plane in a stach of volumes or each rectangle if funct ack."
                    n48 = Index Array(array=w208, index=w207) -> (element=w206:dbl)
                    n49 = Equal To 0?(x=w206) -> (x = 0?=w212:bool)
                    n50 = disable-structure shown="Enabled" {
                      disable-tunnel: w222 -> [w239 _]
                      disable-tunnel: w221 -> [w234 _]
                      disable-tunnel: w220 -> [w232 _]
                      disable-tunnel: w219 -> [w231 _]
                      disable-tunnel: w207 -> [w230 _]
                      disable-tunnel: w218 -> [_ w268]
                      disable-tunnel: w217 -> [_ w267]
                      disable-tunnel: w216 -> [_ w266]
                      disable-tunnel: [_ w265] -> w215
                      disable-tunnel: [_ w264] -> w214
                      disable-tunnel: [_ w263] -> w213
                      disable-tunnel: w212 -> [w229 _]
                      disable-tunnel: w209 -> [w224 w262]
                      disable-tunnel: w211 -> [w227 _]
                      disable-tunnel: w210 -> [w223 _]
                      frame Disabled {
                        # "WARNING!\nUpgrade this code to generate AVI video files instead of individual images.\nUse the code in the \"AVI U16 write-read multi frame.vi\" in C:\\UCL\\RIG 3\\Source Code\\Prototyping\\AVI saves prototyping."
                        n51 = case shown="True" w229 {
                          tunnel: w224 -> [w241 w242]
                          tunnel: [w240 w242] -> w228
                          frame False {
                            # "Vertical"
                            n52 = Transpose 2D Array(2D array=w241) -> (transposed array=w240:u16[][])
                          }
                          frame True {
                            # "Horisontal"
                          }
                        }
                        n53 = call "AVI Video Save.vi"("Image Pixels"=w224) -> ()  [unwired: 9 in, 2 out]
                        n54 = call "IMAQ ArrayToImage"("Image Pixels (I16)"=w228, "Image"=w239) -> ("error out"=w235:errorcluster, "Image Out"=w238:T21)  [unwired: 8 in]
                        n55 = Concatenate Strings(w227, "1" ("string")) -> (w225:string)
                        n56 = call "Generate volume image path.vi"("Channel to process"=w223, "Volume index"=w232, "Number of planes"=w231, "Plane index (within its volume)"=w230, "Folder path"=w234) -> ("File path"=w233:path)  [unwired: 5 in, 1 out]
                        n57 = disable-structure shown="Enabled" {
                          disable-tunnel: w230 -> [w253 _]
                          disable-tunnel: w238 -> [w252 w261]
                          disable-tunnel: [w251 w261] -> w237
                          disable-tunnel: [w249 w260] -> w236
                          disable-tunnel: w235 -> [w250 w260]
                          disable-tunnel: w225 -> [w248 _]
                          frame Enabled {
                            w255 = T20 1 items=["Grayscale (U8)", "Grayscale (I16)", "Grayscale (SGL)", "Complex (CSG)", "RGB (U32)", "HSL (U32)", "RGB (U64)"] ("Image Type")
                            # "Warning!\n-32767 or -32768??"
                            n58 = Number To Decimal String(number=w253) -> (decimal integer string=w256:string)  [unwired: 1 in]
                            n59 = Concatenate Strings(w248, w256) -> (w257:string)
                            n60 = call "IMAQ Create"("Image Name"=w257, "Image Type"=w255, "error in (no error)"=w250) -> ("New Image"=w258:T21, "error out"=w259:errorcluster)  [unwired: 2 in]
                            n61 = call "IMAQ Add"("Image Src A"=w252, "Constant"=i16 -32768, "Image Dst"=w258, "error in (no error)"=w259) -> ("Image Dst Out"=w251:T21, "error out"=w249:errorcluster)  [unwired: 3 in]
                          }
                          frame Disabled {
                          }
                        }
                        n62 = disable-structure shown="Enabled" {
                          disable-tunnel: w237 -> [w245 _]
                          disable-tunnel: w236 -> [w244 _]
                          disable-tunnel: w233 -> [w243 _]
                          frame Enabled {
                            n63 = call-poly "IMAQ Write File 2"("error in (no error)"=w244, "File Path"=w243, "Image"=w245) -> ("error out"=w247:errorcluster, "Image Out (duplicate)"=w246:T21)  [unwired: 7 in]
                            n64 = call "IMAQ Dispose"("Image"=w246, "error in (no error)"=w247) -> ()  [unwired: 4 in, 1 out]
                          }
                          frame Disabled {
                          }
                        }
                      }
                      frame Enabled {
                        # "WARNING!\nPotential issues with this basic implementation can be as follows:\n\n1. It uses the AVI2 implementation which doesn't support generating videos >2GB. \nThe logic would need to be upgraded similarly to the time series imaging code to split the recording into multiple AVI files of <2GB and named suitable.\n\n2. It will place all recorded images in the same AVI file even when they belong to different ROIs like different volumes or different squares.\n\n3. It may error out when ROI sizes differ. To be tested.\nNote to revert to the previous functionality generating individual images simply enable the disabled cases of the 3 yellow structures."
                        n65 = To Unsigned Long Integer(number=w262) -> (unsigned 32bit integer=w270:u32[][])
                        n66 = call "IMAQ ArrayToColorImage"("Image Pixels (U32)"=w270, "Image"=w267, "error in (no error)"=w266) -> ("Image Out"=w271:T21, "error out"=w269:errorcluster)  [unwired: 1 in, 1 out]
                        n67 = call "IMAQ AVI2 Write Frame"("error in (no error)"=w269, "Image"=w271, "AVI Refnum"=w268) -> ("error out"=w265:errorcluster, "Image Out (duplicate)"=w263:T21, "AVI Refnum (duplicate)"=w264:T22)  [unwired: 6 in]
                      }
                    }
                  }
                }
                n68 = disable-structure "Diagram Disable Structure" shown="Enabled" {
                  disable-tunnel: w175 -> [w189 _]
                  disable-tunnel: w178 -> [w188 _]
                  disable-tunnel: w176 -> [w187 _]
                  frame Enabled {
                    n69 = call "IMAQ AVI2 Close"("error in (no error)"=w188, "AVI Refnum"=w189) -> ()  [unwired: 9 in, 1 out]
                    n70 = call "IMAQ Dispose"("Image"=w187) -> ()  [unwired: 5 in, 1 out]
                  }
                  frame Disabled {
                  }
                }
                n71 = call "IMAQ Dispose"("Image"=w177, "error in (no error)"=w178) -> ("error out"=w167:errorcluster)  [unwired: 4 in]
                n72 = flat-sequence {
                  tunnel: w167 -> [w180]
                  tunnel: [w180] -> w166
                  frame #0 {
                    n73 = Request Deallocation(TRUE ("flag")) -> ()
                  }
                }
              }
              frame Error {
              }
            }
          }
        }
      }
    }
    frame Disabled {
      # "The While Loop causes all instances of this VI to execute in parallel. (While loop is REDUNDANT)"
      n74 = while {
        tunnel: [w295] -> w282
        tunnel: w281 -> [w294]
        tunnel: w280 -> [w293]
        tunnel: w279 -> [w289]
        tunnel: w278 -> [w286]
        tunnel: w277 -> [w283]
        stop <- TRUE stop-if-true
        # "The execution speed of this code is not too important as it is run after data acquisition to post-process the TDMS data and pack it into AVI video files which are easier to handle than thousands of individual image files (previously)."
        n75 = call "Reshape volume imaging data.vi"("Channel to process"=w283, "error in (no error)"=w289, "All header parameters"=w286, "TDMS file path & name"=w293) -> ("error out"=w290:errorcluster, "Volumetric parameters"=w284:T19, "Channel 4D data"=w291:u16[][][][], "Angles (deg)"=w285:dbl[])  [unwired: 2 in, 2 out]
        n76 = case shown="\"Green\"" w283 {
          tunnel: ["Red" ("Image Name") "Green" ("Image Name")] -> w292
          tunnel: [Channel_Selector."Red Channel" ("Channel") Channel_Selector."Green Channel" ("Channel")] -> w288
          frame "Red", Default {
            # "Red"
          }
          frame "Green" {
            # "Green"
          }
        }
        n77 = case shown="No Error" w290 {
          selector: w290 -> [_ w408]
          tunnel: [w302 w408] -> w295
          tunnel: w285 -> [w317 _]
          tunnel: w291 -> [w309 _]
          tunnel: w284 -> [w306 _]
          tunnel: w294 -> [w305 _]
          tunnel: w292 -> [w304 _]
          tunnel: w283 -> [w301 _]
          tunnel: w288 -> [w300 _]
          frame No Error {
            w308 = T20 1 items=["Grayscale (U8)", "Grayscale (I16)", "Grayscale (SGL)", "Complex (CSG)", "RGB (U32)", "HSL (U32)", "RGB (U64)", "Grayscale (U16)"] ("Image Type")
            n78 = disable-structure "Diagram Disable Structure" shown="Enabled" {
              disable-tunnel: [w324 _] -> w310
              disable-tunnel: [w323 _] -> w311
              disable-tunnel: [w322 _] -> w312
              disable-tunnel: w305 -> [w321 _]
              disable-tunnel: w300 -> [w320 _]
              frame Enabled {
                n79 = call "Volume acq videos-Initialise.vi"("Channel"=w320, "created path"=w321) -> ("error out"=w324:errorcluster, "Temp Image"=w323:T21, "Refnum out"=w322:T22)  [unwired: 7 in]
              }
              frame Disabled {
              }
            }
            n80 = Unbundle By Name(w306) -> ("number of planes"=w307:i32)
            n81 = call "IMAQ Create"("Image Name"=w304, "Image Type"=w308) -> ("New Image"=w315:T21)  [unwired: 3 in, 1 out]
            n82 = for {
              tunnel: w309 -> [w341] mode=indexing
              tunnel: w315 -> [w340]
              tunnel: w305 -> [w339]
              tunnel: w307 -> [w337]
              tunnel: w311 -> [w336]
              tunnel: w312 -> [w335]
              tunnel: w310 -> [w334]
              tunnel: [w333] -> w316
              tunnel: [w332] -> w313
              tunnel: [w331] -> w314
              tunnel: w317 -> [w330]
              tunnel: w304 -> [w329]
              tunnel: w301 -> [w328]
              i -> [w338]
              # "For each volume in the sequence / Or for each cycle during funct ack."
              n83 = for {
                tunnel: w341 -> [w345] mode=indexing
                tunnel: w340 -> [w358]
                tunnel: w339 -> [w357]
                tunnel: w338 -> [w356]
                tunnel: w337 -> [w355]
                tunnel: w336 -> [w353]
                tunnel: w335 -> [w354]
                tunnel: w334 -> [w352]
                tunnel: [w351] -> w333
                tunnel: [w350] -> w332
                tunnel: [w349] -> w331
                tunnel: w330 -> [w344]
                tunnel: w329 -> [w347]
                tunnel: w328 -> [w346]
                i -> [w343]
                # "For each image/plane in a volume or each rectangle if funct ack."
                n84 = Index Array(array=w344, index=w343) -> (element=w342:dbl)
                n85 = Equal To 0?(x=w342) -> (x = 0?=w348:bool)
                n86 = disable-structure shown="Enabled" {
                  disable-tunnel: w358 -> [w375 _]
                  disable-tunnel: w357 -> [w370 _]
                  disable-tunnel: w356 -> [w368 _]
                  disable-tunnel: w355 -> [w367 _]
                  disable-tunnel: w343 -> [w366 _]
                  disable-tunnel: w354 -> [_ w404]
                  disable-tunnel: w353 -> [_ w403]
                  disable-tunnel: w352 -> [_ w402]
                  disable-tunnel: [_ w401] -> w351
                  disable-tunnel: [_ w400] -> w350
                  disable-tunnel: [_ w399] -> w349
                  disable-tunnel: w348 -> [w365 _]
                  disable-tunnel: w345 -> [w360 w398]
                  disable-tunnel: w347 -> [w363 _]
                  disable-tunnel: w346 -> [w359 _]
                  frame Disabled {
                    # "WARNING!\nUpgrade this code to generate AVI video files instead of individual images.\nUse the code in the \"AVI U16 write-read multi frame.vi\" in C:\\UCL\\RIG 3\\Source Code\\Prototyping\\AVI saves prototyping."
                    n87 = case shown="True" w365 {
                      tunnel: w360 -> [w377 w378]
                      tunnel: [w376 w378] -> w364
                      frame False {
                        # "Vertical"
                        n88 = Transpose 2D Array(2D array=w377) -> (transposed array=w376:u16[][])
                      }
                      frame True {
                        # "Horisontal"
                      }
                    }
                    n89 = call "AVI Video Save.vi"("Image Pixels"=w360) -> ()  [unwired: 9 in, 2 out]
                    n90 = call "IMAQ ArrayToImage"("Image Pixels (I16)"=w364, "Image"=w375) -> ("error out"=w371:errorcluster, "Image Out"=w374:T21)  [unwired: 8 in]
                    n91 = Concatenate Strings(w363, "1" ("string")) -> (w361:string)
                    n92 = call "Generate volume image path.vi"("Channel to process"=w359, "Volume index"=w368, "Number of planes"=w367, "Plane index (within its volume)"=w366, "Folder path"=w370) -> ("File path"=w369:path)  [unwired: 5 in, 1 out]
                    n93 = disable-structure shown="Enabled" {
                      disable-tunnel: w366 -> [w389 _]
                      disable-tunnel: w374 -> [w388 w397]
                      disable-tunnel: [w387 w397] -> w373
                      disable-tunnel: [w385 w396] -> w372
                      disable-tunnel: w371 -> [w386 w396]
                      disable-tunnel: w361 -> [w384 _]
                      frame Enabled {
                        w391 = T20 1 items=["Grayscale (U8)", "Grayscale (I16)", "Grayscale (SGL)", "Complex (CSG)", "RGB (U32)", "HSL (U32)", "RGB (U64)"] ("Image Type")
                        # "Warning!\n-32767 or -32768??"
                        n94 = Number To Decimal String(number=w389) -> (decimal integer string=w392:string)  [unwired: 1 in]
                        n95 = Concatenate Strings(w384, w392) -> (w393:string)
                        n96 = call "IMAQ Create"("Image Name"=w393, "Image Type"=w391, "error in (no error)"=w386) -> ("New Image"=w394:T21, "error out"=w395:errorcluster)  [unwired: 2 in]
                        n97 = call "IMAQ Add"("Image Src A"=w388, "Constant"=i16 -32768, "Image Dst"=w394, "error in (no error)"=w395) -> ("Image Dst Out"=w387:T21, "error out"=w385:errorcluster)  [unwired: 3 in]
                      }
                      frame Disabled {
                      }
                    }
                    n98 = disable-structure shown="Enabled" {
                      disable-tunnel: w373 -> [w381 _]
                      disable-tunnel: w372 -> [w380 _]
                      disable-tunnel: w369 -> [w379 _]
                      frame Enabled {
                        n99 = call-poly "IMAQ Write File 2"("error in (no error)"=w380, "File Path"=w379, "Image"=w381) -> ("error out"=w383:errorcluster, "Image Out (duplicate)"=w382:T21)  [unwired: 7 in]
                        n100 = call "IMAQ Dispose"("Image"=w382, "error in (no error)"=w383) -> ()  [unwired: 4 in, 1 out]
                      }
                      frame Disabled {
                      }
                    }
                  }
                  frame Enabled {
                    # "WARNING!\nPotential issues with this basic implementation can be as follows:\n\n1. It uses the AVI2 implementation which doesn't support generating videos >2GB. \nThe logic would need to be upgraded similarly to the time series imaging code to split the recording into multiple AVI files of <2GB and named suitable.\n\n2. It will place all recorded images in the same AVI file even when they belong to different ROIs like different volumes or different squares.\n\n3. It may error out when ROI sizes differ. To be tested.\nNote to revert to the previous functionality generating individual images simply enable the disabled cases of the 3 yellow structures."
                    n101 = To Unsigned Long Integer(number=w398) -> (unsigned 32bit integer=w406:u32[][])
                    n102 = call "IMAQ ArrayToColorImage"("Image Pixels (U32)"=w406, "Image"=w403, "error in (no error)"=w402) -> ("Image Out"=w407:T21, "error out"=w405:errorcluster)  [unwired: 1 in, 1 out]
                    n103 = call "IMAQ AVI2 Write Frame"("error in (no error)"=w405, "Image"=w407, "AVI Refnum"=w404) -> ("error out"=w401:errorcluster, "Image Out (duplicate)"=w399:T21, "AVI Refnum (duplicate)"=w400:T22)  [unwired: 6 in]
                  }
                }
              }
            }
            n104 = disable-structure "Diagram Disable Structure" shown="Enabled" {
              disable-tunnel: w313 -> [w327 _]
              disable-tunnel: w316 -> [w326 _]
              disable-tunnel: w314 -> [w325 _]
              frame Enabled {
                n105 = call "IMAQ AVI2 Close"("error in (no error)"=w326, "AVI Refnum"=w327) -> ()  [unwired: 9 in, 1 out]
                n106 = call "IMAQ Dispose"("Image"=w325) -> ()  [unwired: 5 in, 1 out]
              }
              frame Disabled {
              }
            }
            n107 = call "IMAQ Dispose"("Image"=w315, "error in (no error)"=w316) -> ("error out"=w303:errorcluster)  [unwired: 4 in]
            n108 = flat-sequence {
              tunnel: w303 -> [w318]
              tunnel: [w318] -> w302
              frame #0 {
                n109 = Request Deallocation(TRUE ("flag")) -> ()
              }
            }
          }
          frame Error {
          }
        }
      }
    }
  }
  "error out" <- w8
  "tdms file out" <- w1
